vi "PC main2.vi"() -> ()   [LabVIEW 2019]
panel:
  in  "stop":bool
  in  "Individual Time[s] 2":dbl
  out "Last J 2":dbl
  out "Numeric 3":i32
  in  "PD Time[s]":dbl
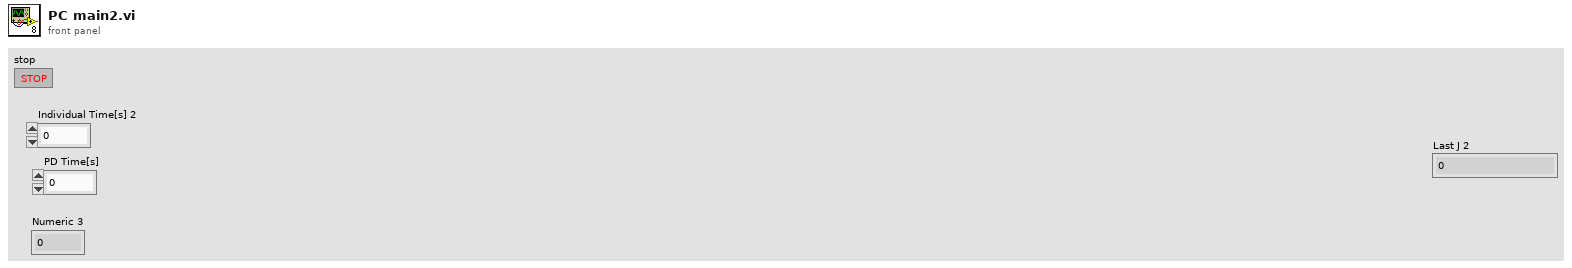
[diagram p1: front panel]
types:
  T1 = enum16{"open", "replace", "create", "open or create", "replace or create", "replace or create with confirmation"}
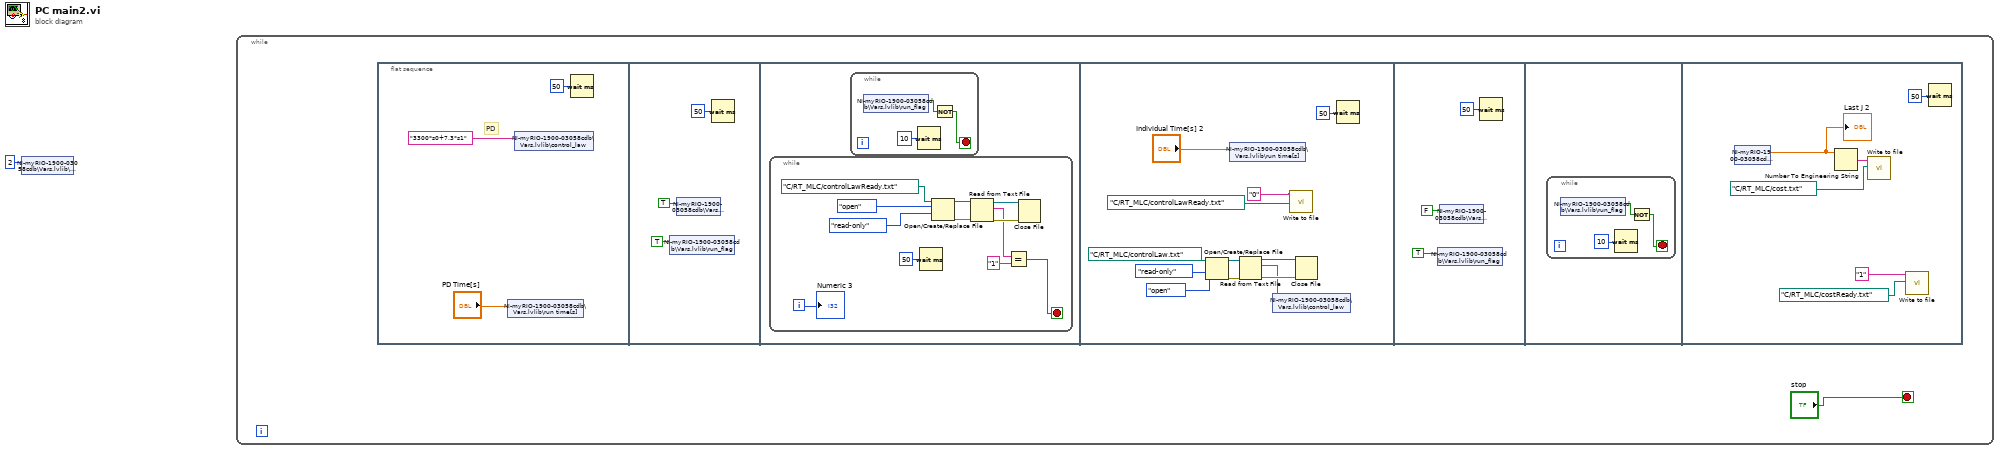
[diagram p0: block diagram]
diagram:
  n1 = shared-variable "NI-myRIO-1900-03058cdb\\Vars.lvlib\\State"(i16 2 ("State")) -> ()  [unwired: 1 in, 1 out]
  n2 = while {
    stop <- "stop" stop-if-true
    n3 = flat-sequence {
      frame #0 {
        # "PD"
        n4 = shared-variable "NI-myRIO-1900-03058cdb\\Vars.lvlib\\run time[s]"("PD Time[s]") -> ()  [unwired: 1 in, 1 out]
        n5 = shared-variable "NI-myRIO-1900-03058cdb\\Vars.lvlib\\control_law"("3300*s0+7.3*s1") -> ()  [unwired: 1 in, 1 out]
        n6 = Wait (ms)(milliseconds to wait=u32 50) -> ()  [unwired: 1 out]
      }
      frame #1 {
        n7 = shared-variable "NI-myRIO-1900-03058cdb\\Vars.lvlib\\run_flag"(TRUE ("run_flag")) -> ()  [unwired: 1 in, 1 out]
        n8 = shared-variable "NI-myRIO-1900-03058cdb\\Vars.lvlib\\PD"(TRUE ("run_flag")) -> ()  [unwired: 1 in, 1 out]
        n9 = Wait (ms)(milliseconds to wait=u32 50) -> ()  [unwired: 1 out]
      }
      frame #2 {
        n10 = while {
          i -> [w13]
          stop <- w12 stop-if-true
          n11 = Wait (ms)(milliseconds to wait=u32 50) -> ()  [unwired: 1 out]
          n12 = Open/Create/Replace File(file path (use dialog)=path "C:/RT_MLC/controlLawReady.txt", operation (0:open)=T1."open", access (0:read/write)=enum16{"read/write", "read-only", "write-only"}."read-only") -> (refnum out=w19:refnum<file>, error out=w20:errorcluster)  [unwired: 3 in, 1 out]
          n13 = Read from Text File(file (use dialog)=w19, error in=w20) -> (refnum out=w21:refnum<file>, text=w14:string, error out=w22:errorcluster)  [unwired: 2 in, 1 out]
          n14 = Equal?(x=w14, y="1") -> (x = y?=w12:bool)
          n15 = Close File(refnum=w21, error in=w22) -> ()  [unwired: 2 out]
          "Numeric 3" <- w13
        }
        n16 = while {
          stop <- w10 stop-if-true
          n17 = shared-variable "NI-myRIO-1900-03058cdb\\Vars.lvlib\\run_flag"() -> (w11:bool)  [unwired: 1 in, 1 out]
          n18 = Wait (ms)(milliseconds to wait=u32 10) -> ()  [unwired: 1 out]
          n19 = Not(x=w11) -> (.not. x?=w10:bool)
        }
      }
      frame #3 {
        n20 = Open/Create/Replace File(file path (use dialog)=path "C:/RT_MLC/controlLaw.txt", operation (0:open)=T1."open", access (0:read/write)=enum16{"read/write", "read-only", "write-only"}."read-only") -> (refnum out=w34:refnum<file>, error out=w35:errorcluster)  [unwired: 3 in, 1 out]
        n21 = shared-variable "NI-myRIO-1900-03058cdb\\Vars.lvlib\\run time[s]"("Individual Time[s] 2") -> ()  [unwired: 1 in, 1 out]
        n22 = Read from Text File(file (use dialog)=w34, error in=w35) -> (refnum out=w29:refnum<file>, text=w28:string, error out=w30:errorcluster)  [unwired: 2 in, 1 out]
        n23 = shared-variable "NI-myRIO-1900-03058cdb\\Vars.lvlib\\control_law"(w28) -> ()  [unwired: 1 in, 1 out]
        n24 = call "Write to file.vi"("file path (use dialog)"=path "C:/RT_MLC/controlLawReady.txt", "String"="0" ("text")) -> ()  [unwired: 10 in]
        n25 = Close File(refnum=w29, error in=w30) -> ()  [unwired: 2 out]
        n26 = Wait (ms)(milliseconds to wait=u32 50) -> ()  [unwired: 1 out]
      }
      frame #4 {
        n27 = shared-variable "NI-myRIO-1900-03058cdb\\Vars.lvlib\\run_flag"(TRUE ("run_flag")) -> ()  [unwired: 1 in, 1 out]
        n28 = shared-variable "NI-myRIO-1900-03058cdb\\Vars.lvlib\\PD"(FALSE ("run_flag")) -> ()  [unwired: 1 in, 1 out]
        n29 = Wait (ms)(milliseconds to wait=u32 50) -> ()  [unwired: 1 out]
      }
      frame #5 {
        n30 = while {
          stop <- w40 stop-if-true
          n31 = shared-variable "NI-myRIO-1900-03058cdb\\Vars.lvlib\\run_flag"() -> (w41:bool)  [unwired: 1 in, 1 out]
          n32 = Wait (ms)(milliseconds to wait=u32 10) -> ()  [unwired: 1 out]
          n33 = Not(x=w41) -> (.not. x?=w40:bool)
        }
      }
      frame #6 {
        n34 = shared-variable "NI-myRIO-1900-03058cdb\\Vars.lvlib\\J"() -> (w46:dbl)  [unwired: 1 in, 1 out]
        "Last J 2" <- w46
        n35 = Number To Engineering String(4:w46) -> (0:w47:string)  [unwired: 3 in]
        n36 = call "Write to file.vi"("file path (use dialog)"=path "C:/RT_MLC/cost.txt", "String"=w47) -> ()  [unwired: 10 in]
        n37 = call "Write to file.vi"("file path (use dialog)"=path "C:/RT_MLC/costReady.txt", "String"="1" ("text")) -> ()  [unwired: 10 in]
        n38 = Wait (ms)(milliseconds to wait=u32 50) -> ()  [unwired: 1 out]
      }
    }
  }
